vi "setEnabledState.vi"(0 "Controller in":refnum<class "_Controller.lvclass">, 1 "state (for single-axis applications only) - (def = DISABLED)":bool, 2 "axes_states (for multi-axis applications only) - (def = DISABLED)":T1, 5 "error in (no error)":errorcluster) -> (14 "Controller out":refnum<class "_Controller.lvclass">, 17 "success?":bool, 18 "response":string, 19 "error out":errorcluster)   [LabVIEW 2020, in "classes.lvlib" / "_Controller.lvclass"]
doc: "If the referenced Arcus controller is single-axis, then the 'state for single-axis applications only' is used to determine enabled/disabled state. If the referenced Arcus controller is multi-axis, then the 'axes_state' input is used.\n\nNOTE: This VI serves as an abstract method to the Controller class. This means it exists for the sole purpose of being overridden by its sub classes (a requirement of the object oriented model).\n\nProduced By:\n\n<B>Kod Integrations, LLC</B>\n4835 Marianne Drive\nMount Airy, MD 21771\nhttp://www.kodintegrations.com\nemail: info@kodintegrations.com\nphone: (240) 687-1288"
uses:
  _Controller.lvclass
  common/controls/motor_enabled_state_axes_group.ctl
  libraries/common.lvlib
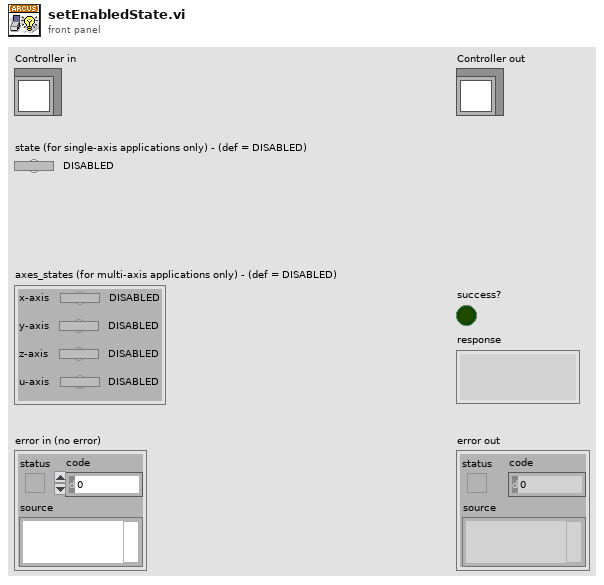
[diagram p1: front panel]
types:
  T1 = typedef "common.lvlib/motor_enabled_state_axes_group.ctl" = cluster{"x-axis":bool, "y-axis":bool, "z-axis":bool, "u-axis":bool}
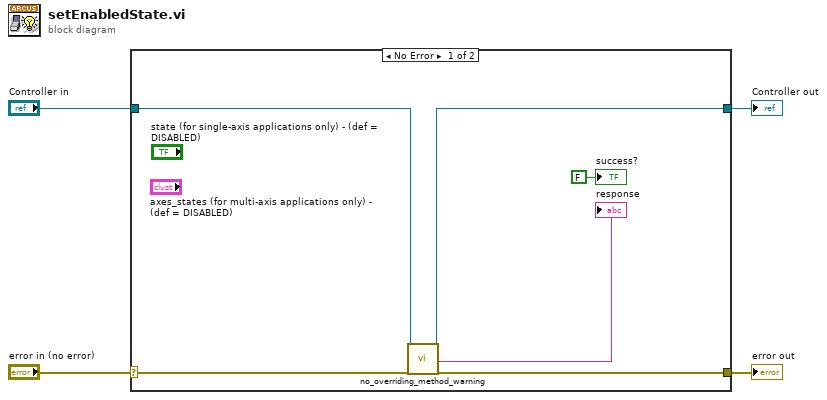
[diagram p0: block diagram]
diagram:
  n1 = case shown="No Error" "error in (no error)" {
    selector: "error in (no error)" -> [w10 w12]
    tunnel: [w9 w12] -> w3
    tunnel: [w7 w11] -> w1
    tunnel: "Controller in" -> [w8 w11]
    frame No Error {
      n2 = call "no_overriding_method_warning.vi"("Controller (in)"=w8, "error in (no error)"=w10) -> ("Controller (out)"=w7:refnum<class "_Controller.lvclass">, "msg"=→"response":string, "error out"=w9:errorcluster)  [unwired: 15 in]
      "success?" <- FALSE ("success?")
    }
    frame Error {
    }
  }
  "error out" <- w3
  "Controller out" <- w1
